vi "Main NR.vi"(8 "error in":errorcluster, 11 "RT Watchdog in":refnum<class "RT Watchdog.lvclass">) -> (0 "error out":errorcluster, 3 "RT Watchdog out":refnum<class "RT Watchdog.lvclass">)   [LabVIEW 2017, in "RT Watchdog.lvclass"]
doc: "The <b>Queued Message Handler</b> of the Worker that owns this VI."
uses:
  RT Watchdog.lvclass
  Initialization Data.ctl
  Response Cases.ctl
  <vilib>/addons/_Workers/Library/Case Label.ctl
  <vilib>/RTwatchdog.llb/Watchdog expiration actions.ctl
  RT Watchdog.lvclass/RT Watchdog.ctl
  rql_Configure Watchdog.ctl
  <vilib>/RTwatchdog.llb/Watchdog status enum.ctl
  rql_Whack Watchdog.ctl
  <vilib>/addons/_Workers/Library/Classes/Message/Priority.ctl
  <vilib>/Utility/error.llb/Error Cluster From Error Code.vi
  <vilib>/ErrorRing/Error Ring.xnode
  <vilib>/addons/_Workers/Library/Workers.lvlib
  <vilib>/addons/_Workers/Library/Classes/Message/Message.lvclass
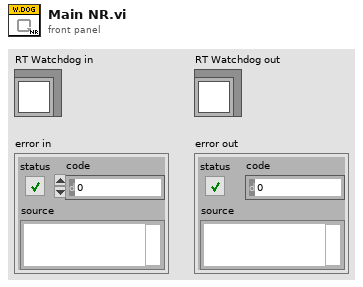
[diagram p1: front panel]
types:
  T1 = typedef "RT Watchdog.lvclass/Initialization Data.ctl" = cluster{"Response Cases":T2, "Debugging Mode?":bool, "expiration actions":T4, "timeout (1 sec)":dbl}
  T2 = typedef "RT Watchdog.lvclass/Response Cases.ctl" = cluster{"Watchdog Expired":T3}
  T3 = typedef "Workers.lvlib/Case Label.ctl" = string
  T4 = typedef "Watchdog expiration actions.ctl" = cluster{"reset system":bool, "restart LabVIEW Runtime":bool, "occurrence":bool, "trigger protocol":enum16{"active high", "active low", "open collector"}, "trigger line":enum16{"none", "line 0", "line 1", "line 2", "line 3", "line 4", "line 5", "line 6", "line 7", "SMB line 0"}, "disable watchdog on VI exit":bool}
  T5 = typedef "Watchdog status enum.ctl" = enum16{"disabled", "expired", "running"}
  T6 = typedef "RT Watchdog.lvclass/rql_Configure Watchdog.ctl" = cluster{"String":string}
  T7 = typedef "RT Watchdog.lvclass/rql_Whack Watchdog.ctl" = cluster{"String":string}
  T8 = typedef "Workers.lvlib/Message.lvclass/Priority.ctl" = enum16{"Low", "Normal", "High"}
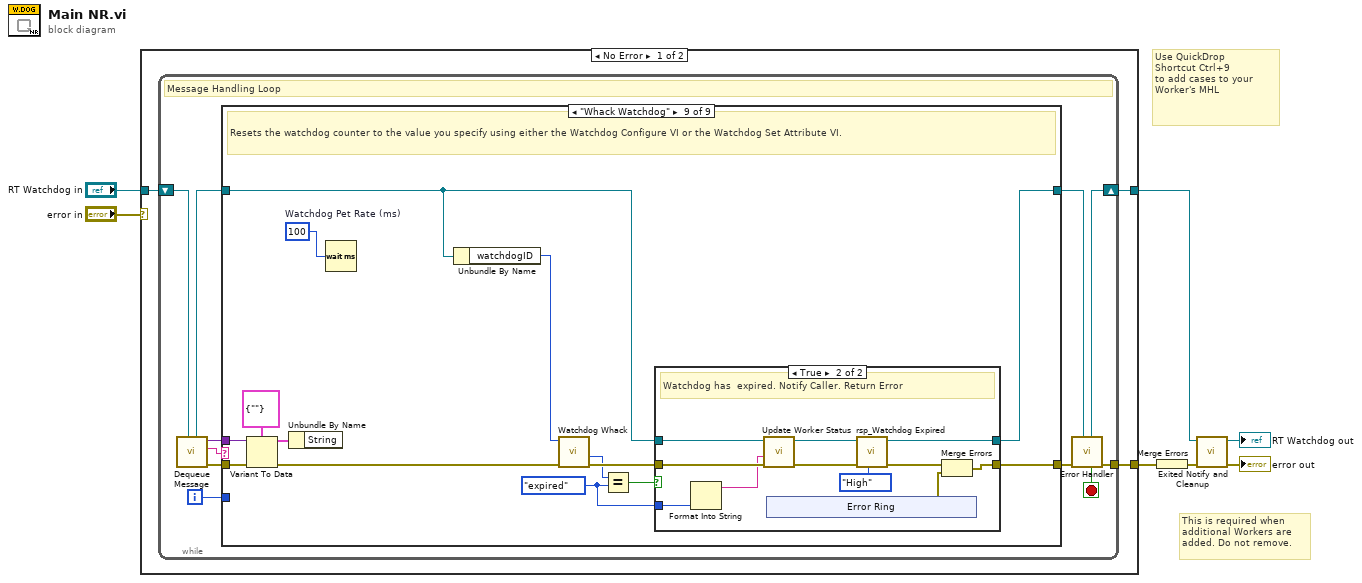
[diagram p0: block diagram]
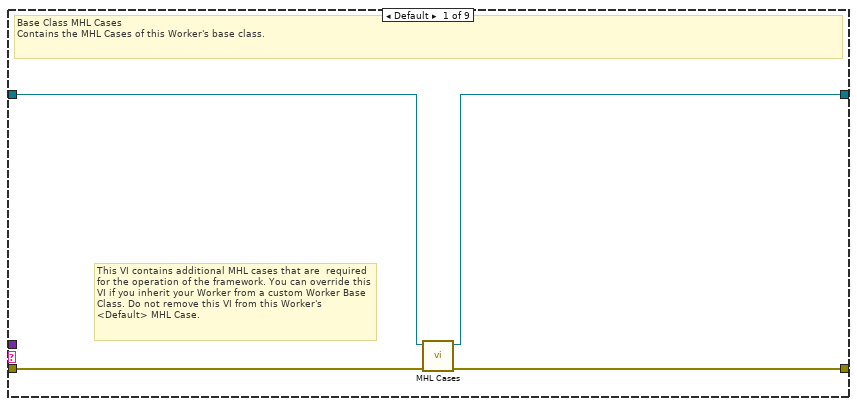
[diagram p2: hidden frame]
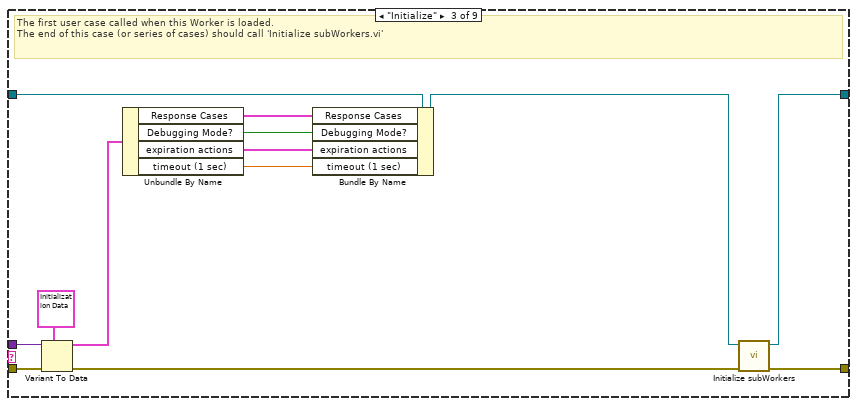
[diagram p4: hidden frame]
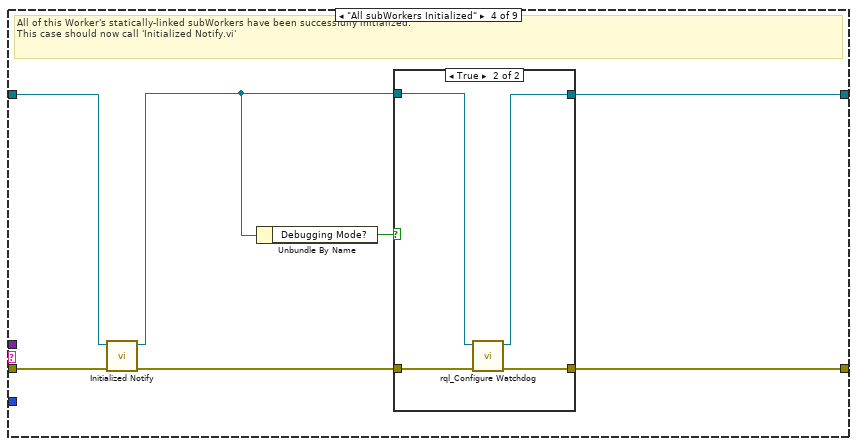
[diagram p5: hidden frame]
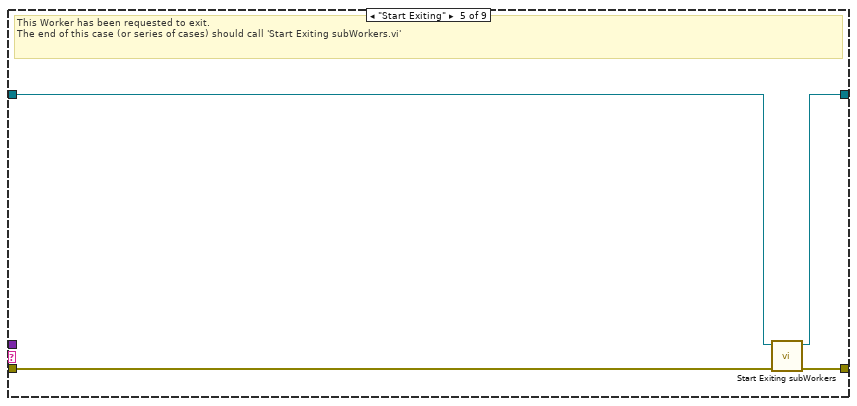
[diagram p7: hidden frame]
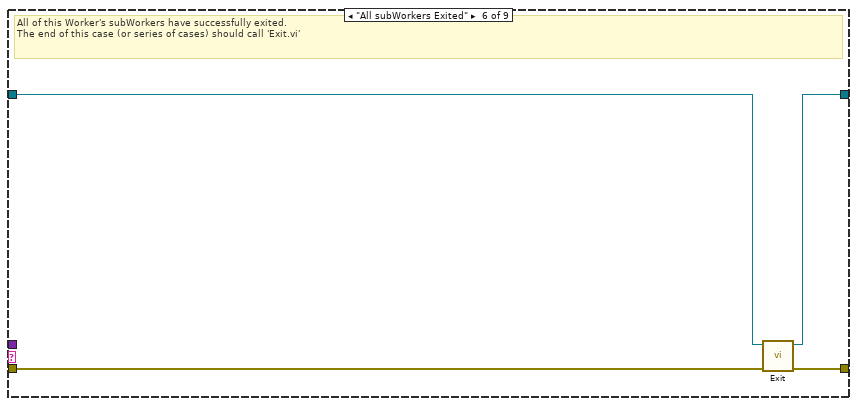
[diagram p8: hidden frame]
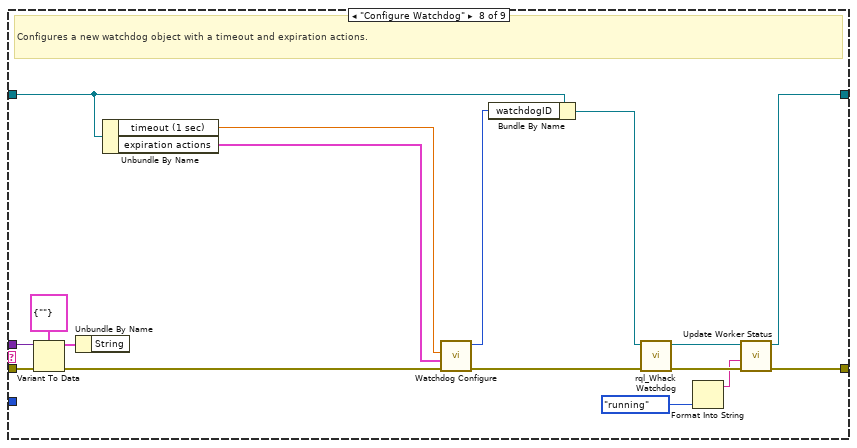
[diagram p10: hidden frame]
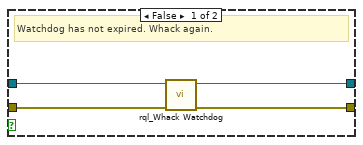
[diagram p11: hidden frame]
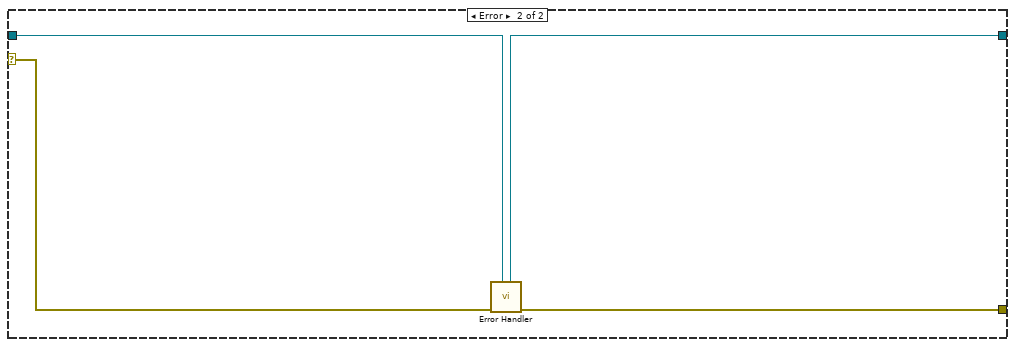
[diagram p12: hidden frame]
diagram:
  # "Use QuickDrop\nShortcut Ctrl+9\nto add cases to your\nWorker's MHL"
  # "This is required when additional Workers are added. Do not remove."
  n1 = case shown="No Error" "error in" {
    tunnel: "RT Watchdog in" -> [w8 w116]
    tunnel: [w10 w117] -> w6
    tunnel: [w9 w115] -> w7
    selector: "error in" -> [_ w118]
    frame No Error {
      n2 = while {
        shift-right: [w19] -> w9
        shift-left: w8 -> [w21]
        tunnel: [w20] -> w10
        i -> [w12]
        stop <- w13 stop-if-true
        # "Message Handling Loop"
        n3 = call-dynamic "Dequeue Message.vi"("Worker"=w21) -> ("error out"=w18:errorcluster, "Case out"=w14:string, "Data out"=w11:variant, "Worker out"=w16:refnum<class "RT Watchdog.lvclass">)  [unwired: 6 in, 1 out]
        n4 = case "Worker MHL Case Structure (DO NOT CHANGE LABEL NAME)" shown="\"Whack Watchdog\"" w14 {
          tunnel: w18 -> [w25 w26 w38 w47 w54 w61 w63 w80 w94]
          tunnel: [w24 w26 w40 w44 w57 w60 w63 w71 w86] -> w17
          tunnel: w16 -> [w23 w27 w33 w45 w55 w59 w62 w66 w85]
          tunnel: [w22 w27 w39 w43 w56 w58 w62 w69 w84] -> w15
          tunnel: w12 -> [_ _ _ _ _ _ _ _ _]
          tunnel: w11 -> [_ _ w36 _ _ _ _ w78 w92]
          frame Default {
            # "This VI contains additional MHL cases that are  required for the operation of the framework. You can override this VI if you inherit your Worker from a custom Worker Base Class. Do not remove this VI from this Worker's <Default> MHL Case."
            # "Base Class MHL Cases\nContains the MHL Cases of this Worker's base class."
            n5 = call-dynamic "MHL Cases.vi"("error in"=w25, "Worker in"=w23) -> ("error out"=w24:errorcluster, "Worker out"=w22:refnum<class "RT Watchdog.lvclass">)  [unwired: 8 in]
          }
          frame "------------ FRAMEWORK CASES -----------" {
            # "Start of Workers Framework Cases"
          }
          frame "Initialize" {
            # "The first user case called when this Worker is loaded.\nThe end of this case (or series of cases) should call 'Initialize subWorkers.vi'"
            n6 = Variant To Data(error in=w38, type=T1 {"Response Cases"={"Watchdog Expired"=""}, "Debugging Mode?"=FALSE, "expiration actions"={"reset system"=FALSE, "restart LabVIEW Runtime"=FALSE, "occurrence"=FALSE, "trigger protocol"=enum."active high", "trigger line"=enum."none", "disable watchdog on VI exit"=TRUE}, "timeout (1 sec)"=1.0} ("Cluster"), Variant=w36) -> (data=w34:T1, error out=w37:errorcluster)
            n7 = Unbundle By Name(w34) -> ("Response Cases"=w35:T2, "Debugging Mode?"=w30:bool, "expiration actions"=w29:T4, "timeout (1 sec)"=w28:dbl)
            n8 = Bundle By Name(cluster=w33, "Response Cases"=w35, "Debugging Mode?"=w30, "expiration actions"=w29, "timeout (1 sec)"=w28) -> (w32:refnum<class "RT Watchdog.lvclass">)
            n9 = call-dynamic "Initialize subWorkers.vi"("error in"=w37, "Worker"=w32) -> ("error out"=w40:errorcluster, "dup Worker out"=w39:refnum<class "RT Watchdog.lvclass">)  [unwired: 8 in]
          }
          frame "All subWorkers Initialized" {
            # "All of this Worker's statically-linked subWorkers have been successfully initialized.\nThis case should now call 'Initialized Notify.vi'"
            n10 = call-dynamic "Initialized Notify.vi"("error in"=w47, "Worker"=w45) -> ("error out"=w46:errorcluster, "dup Worker out"=w42:refnum<class "RT Watchdog.lvclass">)  [unwired: 8 in]
            n11 = Unbundle By Name(w42) -> ("Debugging Mode?"=w41:bool)
            n12 = case shown="True" w41 {
              tunnel: w46 -> [w48 w53]
              tunnel: [w48 w52] -> w44
              tunnel: w42 -> [w49 w51]
              tunnel: [w49 w50] -> w43
              frame False {
                # "Do not enable the watchdog when debugging."
              }
              frame True {
                n13 = call "rql_Configure Watchdog.vi"("error in"=w53, "RT Watchdog in"=w51) -> ("error out"=w52:errorcluster, "dup RT Watchdog out"=w50:refnum<class "RT Watchdog.lvclass">)  [unwired: 8 in]
              }
            }
          }
          frame "Start Exiting" {
            # "This Worker has been requested to exit. \nThe end of this case (or series of cases) should call 'Start Exiting subWorkers.vi'"
            n14 = call-dynamic "Start Exiting subWorkers.vi"("error_in"=w54, "Worker"=w55) -> ("error out"=w57:errorcluster, "dup Worker out"=w56:refnum<class "RT Watchdog.lvclass">)  [unwired: 8 in]
          }
          frame "All subWorkers Exited" {
            # "All of this Worker's subWorkers have successfully exited. \nThe end of this case (or series of cases) should call 'Exit.vi'"
            n15 = call-dynamic "Exit.vi"("error_in"=w61, "Worker"=w59) -> ("error out"=w60:errorcluster, "dup Worker out"=w58:refnum<class "RT Watchdog.lvclass">)  [unwired: 8 in]
          }
          frame "------------- LOCAL API CASES -------------" {
            # "Start of Workers Local API Cases"
          }
          frame "Configure Watchdog" {
            # "Configures a new watchdog object with a timeout and expiration actions."
            n16 = Variant To Data(error in=w80, type=T6 {"String"=""} ("Data"), Variant=w78) -> (data=w77:T6, error out=w76:errorcluster)
            n17 = Unbundle By Name(w77) -> ()  [unwired: 1 out]
            n18 = Unbundle By Name(w66) -> ("timeout (1 sec)"=w65:dbl, "expiration actions"=w64:T4)
            n19 = call <vilib>:"Watchdog Configure.vi"("error in (no error)"=w76, "expiration actions"=w64, "timeout (1 sec)"=w65) -> ("error out"=w75:errorcluster, "watchdogID"=w74:u64)  [unwired: 1 in, 2 out]
            n20 = Bundle By Name(cluster=w66, "watchdogID"=w74) -> (w72:refnum<class "RT Watchdog.lvclass">)
            n21 = call "rql_Whack Watchdog.vi"("error in"=w75, "RT Watchdog in"=w72) -> ("error out"=w73:errorcluster, "dup RT Watchdog out"=w70:refnum<class "RT Watchdog.lvclass">)  [unwired: 8 in]
            n22 = Format Into String(Watchdog_status_enum."running" ("watchdog status")) -> (resulting string=w67:string)  [unwired: 3 in, 1 out]
            n23 = call-dynamic "Update Worker Status.vi"("error in"=w73, "Worker Status"=w67, "Worker"=w70) -> ("error out"=w71:errorcluster, "dup Worker out"=w69:refnum<class "RT Watchdog.lvclass">)  [unwired: 7 in]
          }
          frame "Whack Watchdog" {
            w81 = Watchdog_status_enum."expired" ("watchdog status")
            w87 = u32 100  # Watchdog Pet Rate (ms)
            # "Resets the watchdog counter to the value you specify using either the Watchdog Configure VI or the Watchdog Set Attribute VI."
            n24 = Variant To Data(error in=w94, type=T7 {"String"=""} ("Data"), Variant=w92) -> (data=w91:T7, error out=w90:errorcluster)
            n25 = Unbundle By Name(w91) -> ()  [unwired: 1 out]
            n26 = Wait (ms)(milliseconds to wait=w87) -> ()  [unwired: 1 out]
            n27 = Unbundle By Name(w85) -> ("watchdogID"=w88:u64)
            n28 = call <vilib>:"Watchdog Whack.vi"("error in (no error)"=w90, "watchdogID in"=w88) -> ("error out"=w89:errorcluster, "watchdog status"=w83:T5)  [unwired: 3 in, 1 out]
            n29 = Equal?(x=w83, y=w81) -> (x = y?=w82:bool)
            n30 = case shown="True" w82 {
              tunnel: w89 -> [w98 w109]
              tunnel: [w97 w104] -> w86
              tunnel: w85 -> [w96 w107]
              tunnel: [w95 w100] -> w84
              tunnel: w81 -> [_ w106]
              frame False {
                # "Watchdog has not expired. Whack again."
                n31 = call "rql_Whack Watchdog.vi"("error in"=w98, "RT Watchdog in"=w96) -> ("error out"=w97:errorcluster, "dup RT Watchdog out"=w95:refnum<class "RT Watchdog.lvclass">)  [unwired: 8 in]
              }
              frame True {
                # "Watchdog has  expired. Notify Caller. Return Error"
                n32 = Format Into String(w106) -> (resulting string=w105:string)  [unwired: 3 in, 1 out]
                n33 = call-dynamic "Update Worker Status.vi"("error in"=w109, "Worker Status"=w105, "Worker"=w107) -> ("error out"=w108:errorcluster, "dup Worker out"=w101:refnum<class "RT Watchdog.lvclass">)  [unwired: 7 in]
                n34 = xnode "Error Ring"() -> ("error out"=w103:errorcluster)
                n35 = call "rsp_Watchdog Expired.vi"("Message Priority"=Priority."High", "error in"=w108, "RT Watchdog in"=w101) -> ("error out"=w102:errorcluster, "dup RT Watchdog out"=w100:refnum<class "RT Watchdog.lvclass">)  [unwired: 7 in]
                n36 = Merge Errors(w102, w103) -> (w104:errorcluster)
              }
            }
          }
        }
        n37 = call-dynamic "Error Handler.vi"("Worker"=w15, "error_in"=w17) -> ("error out"=w20:errorcluster, "Stop Loop"=w13:bool, "Worker out"=w19:refnum<class "RT Watchdog.lvclass">)  [unwired: 7 in]
      }
    }
    frame Error {
      n38 = call-dynamic "Error Handler.vi"("Worker"=w116, "error_in"=w118) -> ("error out"=w117:errorcluster, "Worker out"=w115:refnum<class "RT Watchdog.lvclass">)  [unwired: 7 in, 1 out]
    }
  }
  n39 = Merge Errors(w6) -> (w3:errorcluster)
  n40 = call-dynamic "Exited Notify and Cleanup.vi"("error_in"=w3, "Worker"=w7) -> ("error out"=→"error out":errorcluster, "dup Worker out"=→"RT Watchdog out":refnum<class "RT Watchdog.lvclass">)  [unwired: 8 in]
